vi "to string.vi"(8 "error in":errorcluster, 11 "Standard Engine Repo Data in":refnum<class "Standard Engine Configuration.lvclass">) -> (0 "error out":errorcluster, 1 "data":string, 2 "version":string, 3 "Standard Engine Repo Data out":refnum<class "Standard Engine Configuration.lvclass">)   [LabVIEW 2013, in "Standard Engine Configuration.lvclass"]
uses:
  Standard Engine Configuration.lvclass
  <vilib>/NI/Module Execution Interface/Engine Configuration/engine configuration.lvclass
  Standard Engine Configuration.lvclass/Standard Engine Configuration.ctl
  <vilib>/NI/Tag Bus Module Framework/root configuration/TBM configuration.lvclass
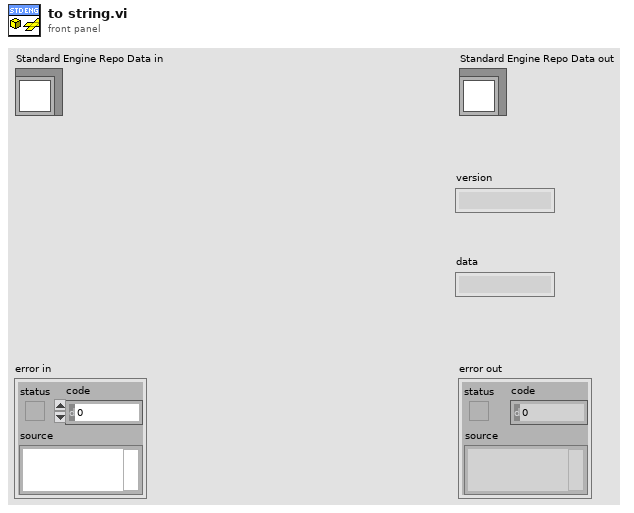
[diagram p1: front panel]
types:
  T1 = typedef "Standard Engine Configuration.lvclass/Engine Configuration.ctl" = cluster{"Loop Info":T2, "Timing Source Type":T3, "Timing Source dt":u32, "Master Timing Module":string, "Module Specific Configuration":T4[]}
  T2 = typedef "Standard Engine Configuration.lvclass/Loop Info.ctl" = cluster{"Processor":i32, "Priority":i32}
  T3 = typedef "Standard Engine Configuration.lvclass/Supported Timing Sources.ctl" = enum16{"Use Module Timing Source", "1 kHz Clock", "1 MHz Clock", "Synchronize to Scan Engine"}
  T4 = typedef "Standard Engine Configuration.lvclass/Module Specific Configuration.ctl" = cluster{"Module ID":string, "Module Decimation":T5, "Module Error Configuration":T6}
  T5 = typedef "Standard Engine Configuration.lvclass/Module Decimation.ctl" = cluster{"Decimation":u16, "Offset":u16}
  T6 = typedef "Standard Engine Configuration.lvclass/Module Error Configuration.ctl" = cluster{"Module Error Configuration":T7[]}
  T7 = typedef "Standard Engine Configuration.lvclass/Error Actions By Category.ctl" = cluster{"error classification":T8, "Error Actions":T9[]}
  T8 = typedef "TBM module execution interface.lvclass/error classification.ctl" = enum16{"unknown", "none", "trivial", "recoverable", "critical"}
  T9 = typedef "Standard Engine Configuration.lvclass/Error Actions.ctl" = enum16{"Clear", "Notify", "Stop Component", "Stop Engine", "Safe State", "Attempt Recovery"}
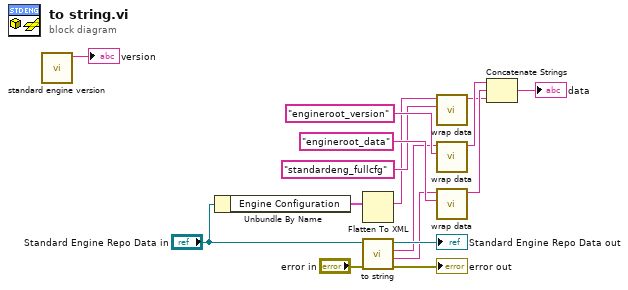
[diagram p0: block diagram]
diagram:
  n1 = call "standard engine version.vi"() -> ("Version"=→"version":string)  [unwired: 11 in]
  n2 = Unbundle By Name("Standard Engine Repo Data in") -> ("Engine Configuration"=w2:T1)
  n3 = Flatten To XML(anything=w2) -> (xml string=w3:string)
  n4 = call-parent "to string.vi"("error in"="error in", "engine configuration in"="Standard Engine Repo Data in") -> ("error out"=→"error out":errorcluster, "data"=w5:string, "version"=w6:string, "engine configuration out"=→"Standard Engine Repo Data out":refnum<class "Standard Engine Configuration.lvclass">)  [unwired: 6 in]
  n5 = call <vilib>:"wrap data.vi"("identifier"="standardeng_fullcfg" ("additional identifier"), "data to wrap"=w3) -> ("wrapped data"=w7:string)  [unwired: 9 in]
  n6 = call <vilib>:"wrap data.vi"("identifier"="engineroot_version" ("additional identifier"), "data to wrap"=w6) -> ("wrapped data"=w9:string)  [unwired: 9 in]
  n7 = call <vilib>:"wrap data.vi"("identifier"="engineroot_data" ("additional identifier"), "data to wrap"=w5) -> ("wrapped data"=w10:string)  [unwired: 9 in]
  n8 = Concatenate Strings(w9, w10, w7) -> (→"data":string)
